vi "Message.vi"(2 "Enum":enum16{"Error", "Warning", "OK"}(ring), 3 "error in (no error)":errorcluster, 5 "Message":string) -> (0 "error out":errorcluster, 1 "Ok 2":bool)   [LabVIEW 2017]
doc: "Update message on display."
panel:
  in  "Ok":bool
  out "Message":string
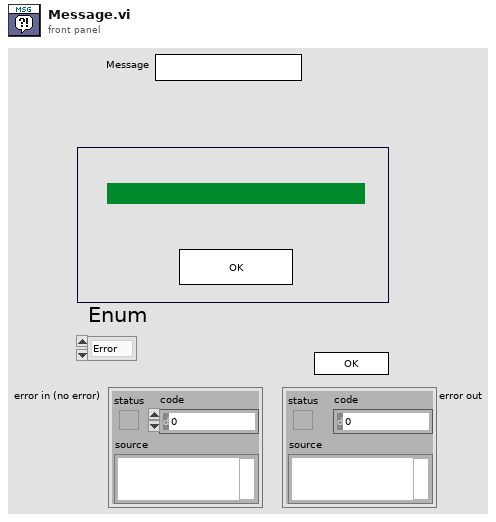
[diagram p1: front panel]
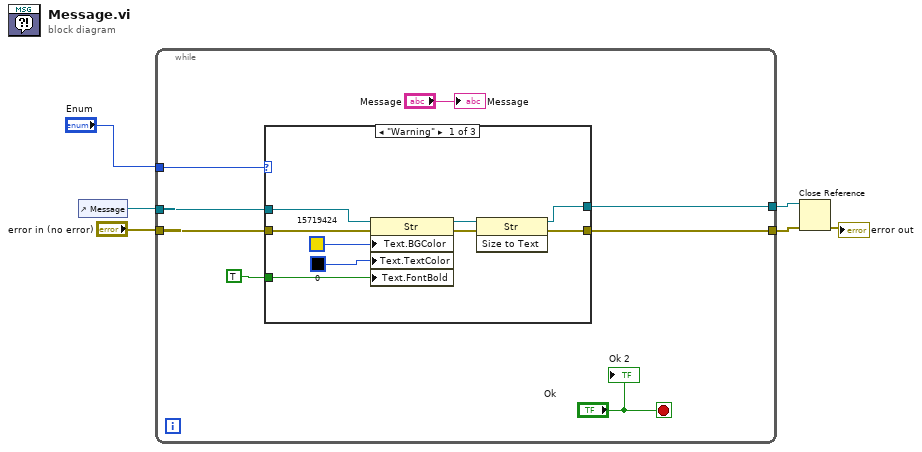
[diagram p0: block diagram]
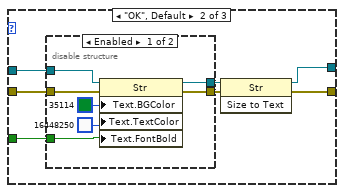
[diagram p2: hidden frame]
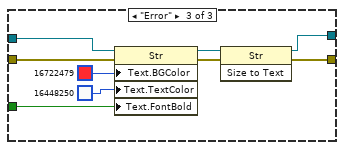
[diagram p4: hidden frame]
diagram:
  n1 = control-ref of="Message"() -> (w5:refnum<vi>)
  n2 = while {
    tunnel: "error in (no error)" -> [w11]
    tunnel: [w10] -> w4
    tunnel: w5 -> [w12]
    tunnel: [w9] -> w3
    tunnel: "Enum" -> [w8]
    stop <- "Ok" stop-if-true
    n3 = case shown="\"Warning\"" w8 {
      tunnel: w12 -> [w19 w26 w45]
      tunnel: w11 -> [w21 w28 w46]
      tunnel: [w23 w30 w48] -> w10
      tunnel: [w22 w29 w47] -> w9
      tunnel: TRUE -> [w15 w24 w40]
      frame "Warning" {
        n4 = property class="Str"(reference=w19, error in=w21, "Text.BGColor"=u32 15719424, "Text.TextColor"=u32 0, "Text.FontBold"=w15) -> (reference out=w18:refnum<vi>, error out=w20:errorcluster)
        n5 = invoke class="Str" method="Size to Text"(reference=w18, error in=w20) -> (reference out=w22:refnum<vi>, error out=w23:errorcluster)  [unwired: 1 in, 1 out]
      }
      frame "OK", Default {
        n6 = disable-structure shown="Enabled" {
          disable-tunnel: w28 -> [w37 w39]
          disable-tunnel: [w36 w39] -> w27
          disable-tunnel: w26 -> [w35 w38]
          disable-tunnel: [w34 w38] -> w25
          disable-tunnel: w24 -> [w31 _]
          frame Enabled {
            n7 = property class="Str"(reference=w35, error in=w37, "Text.BGColor"=u32 35114, "Text.TextColor"=u32 16448250, "Text.FontBold"=w31) -> (reference out=w34:refnum<vi>, error out=w36:errorcluster)
          }
          frame Disabled {
          }
        }
        n8 = invoke class="Str" method="Size to Text"(reference=w25, error in=w27) -> (reference out=w29:refnum<vi>, error out=w30:errorcluster)  [unwired: 1 in, 1 out]
      }
      frame "Error" {
        n9 = property class="Str"(reference=w45, error in=w46, "Text.BGColor"=u32 16722479, "Text.TextColor"=u32 16448250, "Text.FontBold"=w40) -> (reference out=w43:refnum<vi>, error out=w44:errorcluster)
        n10 = invoke class="Str" method="Size to Text"(reference=w43, error in=w44) -> (reference out=w47:refnum<vi>, error out=w48:errorcluster)  [unwired: 1 in, 1 out]
      }
    }
    "Message" <- "Message"
    "Ok 2" <- "Ok"
  }
  n11 = Close Reference(reference=w3, error in (no error)=w4) -> (error out=→"error out":errorcluster)
